vi "闹钟（时分秒）.vi"(5 "设定时分秒":i32 format="%< %H-%M-%S>t", 7 "启用":bool=TRUE) -> (6 "时间到脉冲":bool, 8 "当前时分秒":i32 format="%< %H-%M-%S>t")   [LabVIEW 2012]
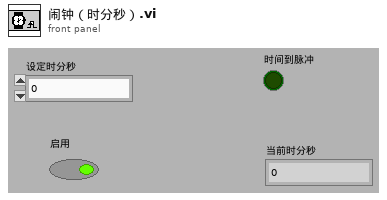
[diagram p1: front panel]
types:
  T1 = typedef "LVDateTimeRec.ctl" = cluster{"秒数的小数部分":dbl, "秒":i32, "分":i32, "时":i32, "日":i32, "月":i32, "年":i32, "天数（周）":i32, "天数（年）":i32, "DST":i32}
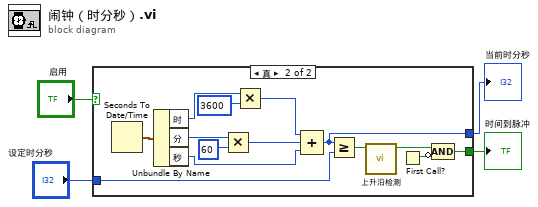
[diagram p0: block diagram]
diagram:
  n1 = case shown="真" "启用" {
    tunnel: "设定时分秒" -> [_ w15]
    tunnel: [_ w17] -> w3
    tunnel: [_ w5] -> w2
    frame False {
    }
    frame True {
      n2 = Seconds To Date/Time() -> (date time rec=w18:T1)  [unwired: 2 in]
      n3 = Unbundle By Name(w18) -> ("时"=w12:i32, "分"=w10:i32, "秒"=w6:i32)
      n4 = Multiply(x=w10, y=60) -> (x*y=w8:i32)
      n5 = Multiply(x=w12, y=3600) -> (x*y=w7:i32)
      n6 = Compound Arithmetic op=ADD(w7, w8, w6) -> (w5:i32)
      n7 = Greater Or Equal?(x=w5, y=w15) -> (x >= y?=w14:bool)
      n8 = call "上升沿检测.vi"("input"=w14) -> ("output"=w13:bool)  [unwired: 9 in, 1 out]
      n9 = First Call?() -> (First Call?: T/F=w16:bool)
      n10 = Compound Arithmetic op=AND(w13, invert w16) -> (w17:bool)
    }
  }
  "时间到脉冲" <- w3
  "当前时分秒" <- w2
